vi "create_trajectory.vi"(8 "error in (no error)":errorcluster, 11 "anchor points":refnum<class "SpaceVector.lvclass">[](array[class])) -> (0 "error out":errorcluster)   [LabVIEW 2010]
uses:
  SpaceVector.lvclass
panel:
  in  "divisor":dbl=1.0
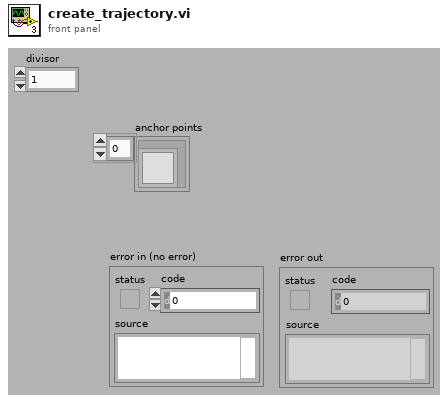
[diagram p1: front panel]
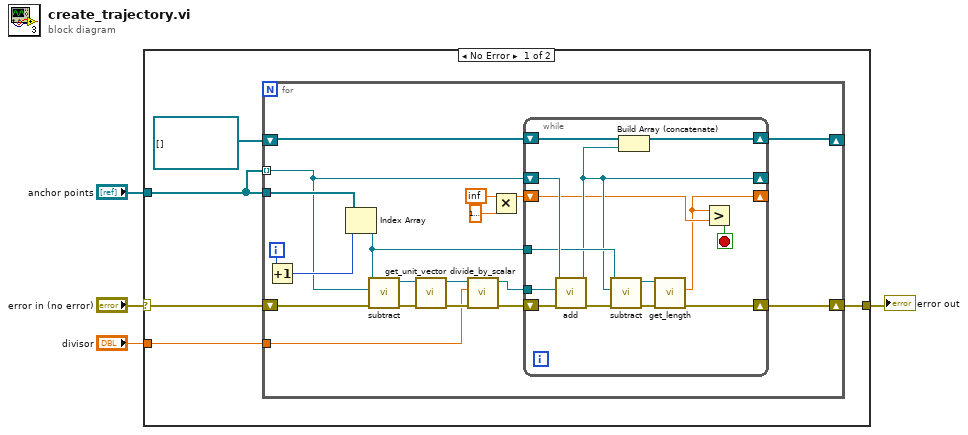
[diagram p0: block diagram]
diagram:
  n1 = case shown="No Error" "error in (no error)" {
    selector: "error in (no error)" -> [w8 w43]
    tunnel: "anchor points" -> [w5 _]
    tunnel: [w9 w43] -> w2
    tunnel: "divisor" -> [w7 _]
    frame No Error {
      n2 = for {
        tunnel: w5 -> [w27]
        tunnel: w7 -> [w20]
        shift-right: [w28] -> w9
        shift-left: w8 -> [w26]
        shift-right: [w12] -> _
        shift-left: refnum<class "SpaceVector.lvclass">[] [] -> [w11]
        tunnel: w5 -> [w10] mode=indexing
        i -> [w18]
        n3 = Increment(x=w18) -> (x+1=w17:i32)
        n4 = Index Array(array=w27, index=w17) -> (element=w16:refnum<class "SpaceVector.lvclass">)
        n5 = call "subtract.vi"("error in (no error)"=w26, "subtrahend"=w10, "SpaceVector in"=w16) -> ("error out"=w24:errorcluster, "SpaceVector out"=w25:refnum<class "SpaceVector.lvclass">)  [unwired: 7 in]
        n6 = call "get_unit_vector.vi"("error in (no error)"=w24, "SpaceVector in"=w25) -> ("error out"=w23:errorcluster, "SpaceVector out"=w22:refnum<class "SpaceVector.lvclass">)  [unwired: 7 in, 1 out]
        n7 = call "divide_by_scalar.vi"("error in (no error)"=w23, "divisor"=w20, "SpaceVector in"=w22) -> ("error out"=w21:errorcluster, "SpaceVector out"=w19:refnum<class "SpaceVector.lvclass">)  [unwired: 7 in]
        n8 = Multiply(x=inf, y=dbl[unit] 1e-06) -> (x*y=w14:dbl[unit])
        n9 = while {
          shift-right: [w33] -> w28
          shift-left: w21 -> [w42]
          shift-right: [w36] -> _
          shift-left: w10 -> [w41]
          tunnel: w19 -> [w40]
          shift-right: [w38] -> w12
          shift-left: w11 -> [w39]
          tunnel: w16 -> [w37]
          shift-right: [w29] -> _
          shift-left: w14 -> [w31]
          stop <- w30 stop-if-true
          n10 = call "add.vi"("error in (no error)"=w42, "vector to be added"=w40, "SpaceVector in"=w41) -> ("error out"=w35:errorcluster, "SpaceVector out"=w36:refnum<class "SpaceVector.lvclass">)  [unwired: 7 in]
          n11 = call "subtract.vi"("error in (no error)"=w35, "subtrahend"=w36, "SpaceVector in"=w37) -> ("error out"=w34:errorcluster, "SpaceVector out"=w32:refnum<class "SpaceVector.lvclass">)  [unwired: 7 in]
          n12 = Build Array (concatenate)(w39, w36) -> (w38:refnum<class "SpaceVector.lvclass">[])
          n13 = call "get_length.vi"("error in (no error)"=w34, "SpaceVector in"=w32) -> ("error out"=w33:errorcluster, "length"=w29:dbl[unit])  [unwired: 7 in, 1 out]
          n14 = Greater?(x=w29, y=w31) -> (0:w30:bool)
        }
      }
    }
    frame Error {
    }
  }
  "error out" <- w2
